vi "Set jog parameters.vi"(0 "Resource":refnum<k21>="nism://My Computer/Axis 1") -> (1 "resource out":refnum<k21>, 2 "Current position [deg]":dbl format="%0.0f", 3 "Jog position setting [deg]":dbl, 4 "Jog velocity setting [rev/s]":dbl, 5 "Start jog setting":bool, 6 "Jog complete setting":bool)   [LabVIEW 2018]
uses:
  <vilib>/Motion/Express/_s/nimc.ex.resetPosition.resetPosition.axis.vi
  <vilib>/Motion/Express/_s/nimc.ex.read.readExecutionData.axis.vi
  <vilib>/Motion/BlockNode/FB.NIMotion.xnode
  <vilib>/ptbypt/NI_PtbyPt.lvlib
panel:
  in  "Reset motor position":bool
  in  "Next Button":bool
  in  "OK Button":bool
  in  "Jog velocity [rev/s]":dbl format="%#_1g"
  in  "Jog position [deg]":dbl
  # "Set jog parameters. After 'Start jog' is pressed jog move will begin in selected direction and velocity. Position moves are absolute. Enter positive values for CW rotation, negative for CCW. CCW direction increases load. 'Jog complete' will proceed to states following jog move."
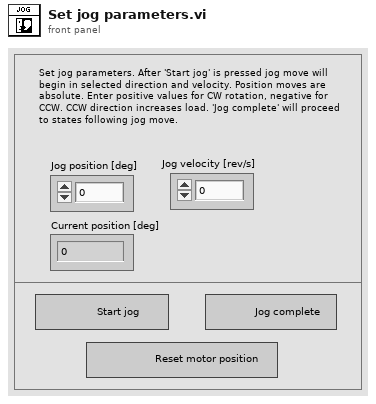
[diagram p1: front panel]
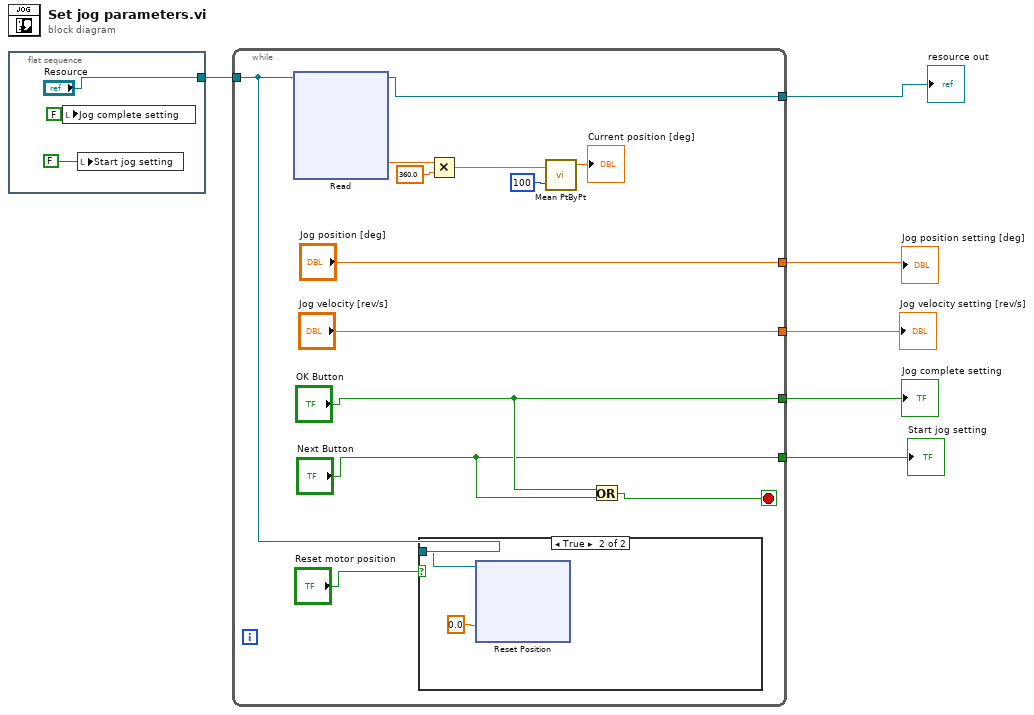
[diagram p0: block diagram]
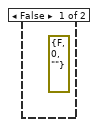
[diagram p2: hidden frame]
diagram:
  n1 = flat-sequence {
    tunnel: ["Resource"] -> w2
    frame #0 {
      n2 = local write "Jog complete setting"(FALSE ("OK Button setting")) -> ()
      n3 = local write "Start jog setting"(FALSE ("Next Button Setting")) -> ()
    }
  }
  n4 = while {
    tunnel: ["Jog position [deg]"] -> w6
    tunnel: ["Jog velocity [rev/s]"] -> w5
    tunnel: ["Next Button"] -> w4
    tunnel: ["OK Button"] -> w3
    tunnel: w2 -> [w10]
    tunnel: [w17] -> w1
    stop <- w19 stop-if-true
    n5 = xnode ("Read")("resource"=w10) -> ("position"=w15:dbl, "resource out"=w17:refnum<k21>)  [unwired: 1 in, 5 out]
    n6 = case shown="True" "Reset motor position" {
      tunnel: w10 -> [_ w23]
      frame False {
        (unwired) errorcluster {"status"=FALSE, "code"=0, "source"=""} ("error out")
      }
      frame True {
        n7 = xnode ("Reset Position")("position"=0.0, "resource"=w23) -> ()  [unwired: 1 in, 2 out]
      }
    }
    n8 = Multiply(x=w15, y=360.0) -> (x*y=w13:dbl)
    n9 = call <vilib>:"Mean PtByPt.vi"("x"=w13, "sample length"=100) -> ("mean"=→"Current position [deg]":dbl)  [unwired: 2 in, 1 out]
    n10 = Or(x="OK Button", y="Next Button") -> (x .or. y?=w19:bool)
  }
  "Jog position setting [deg]" <- w6
  "Jog velocity setting [rev/s]" <- w5
  "Start jog setting" <- w4
  "Jog complete setting" <- w3
  "resource out" <- w1
